vi "Format Class List Table.vi"(5 "Detail Level":T1, 7 "Msg Chain in":string, 8 "error in (no error)":errorcluster, 10 "Class Info Array":T2[](array[typedef]), 11 "VIDoc Printer - Confluence In":refnum<class "VIDoc Printer - Confluence.lvclass">) -> (0 "error out":errorcluster, 2 "Table Text":string, 3 "VIDoc Printer - Confluence Out":refnum<class "VIDoc Printer - Confluence.lvclass">)   [LabVIEW 2023, in "VIDoc Printer - Confluence.lvlib" / "VIDoc Printer - Confluence.lvclass"]
uses:
  VIDoc Printer - Confluence.lvclass
  C:/projects/DMC/Tooling/Git-Action-Service/Source/Documentation Generation/Printers/Printer/VIDoc Printer.lvclass
  Parsing/TypeDefs/Base Class Info Cluster.ctl
  <vilib>/picture/picture.llb/imagedata.ctl
  Settings/Printer Settings/Detail Level Enum.ctl
  VIDoc Printer - Confluence.lvclass/VIDoc Printer - Confluence.ctl
  Accessors/Get Class Column Ordering - Full.vi
  Accessors/Get Class Column Ordering - Minimal.vi
  Accessors/Get Class Column Ordering - Standard.vi
  Accessors/Get Sortable Tables.vi
  Printer/VIDoc Printer.lvclass
  UI Interaction/UI Interaction.lvclass
  Confluence Formatting/Confluence Formatting.lvlib
  C:/projects/DMC/Tooling/Git-Action-Service/Source/Documentation Generation/Printers/Confluence Printer/VIDoc Printer - Confluence.lvclass
  Parsing/VIDoc Parsing.lvlib
  Settings/Printer Settings/Printer Settings.lvclass
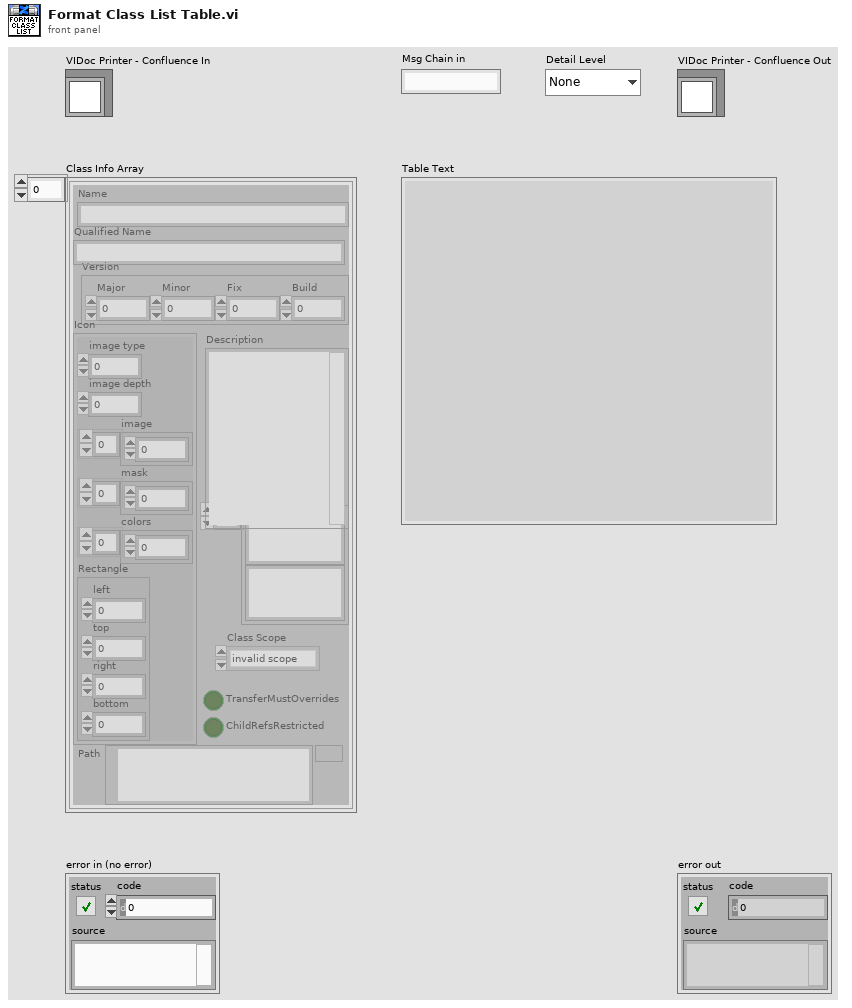
[diagram p1: front panel]
types:
  T1 = typedef "VIDoc Printer.lvlib/Printer Settings.lvclass/Detail Level Enum.ctl" = enum16{"None", "Minimal", "Standard", "Full"}
  T2 = typedef "VIDoc Parsing.lvlib/Base Class Info Cluster.ctl" = cluster{"Name":string, "Icon":T3, "Version":cluster{"Major":u16, "Minor":u16, "Fix":u16, "Build":u16}, "Description":string, "Friends":string[], "ChildRefsRestricted":bool, "TransferMustOverrides":bool, "Path":path, "Qualified Name":string, "Class Scope":enum32{"invalid scope", "public", "private", "protected", "community"}}
  T3 = typedef "imagedata.ctl" = cluster{"image type":i32, "image depth":i32, "image":u8[], "mask":u8[], "colors":u32[], "Rectangle":cluster{"left":i16, "top":i16, "right":i16, "bottom":i16}}
  T4 = cluster{"Major":u16, "Minor":u16, "Fix":u16, "Build":u16}
  T5 = typedef "VIDoc Printer - Confluence.lvlib/VIDoc Settings - Confluence.lvclass/Class Info Column.ctl" = enum16{"Image", "Name", "Description", "Version", "Last Change", "Author", "Commit Hash", "Branch", "Qualified Name", "TransferMustOverrides", "ChildRefsRestricted"}
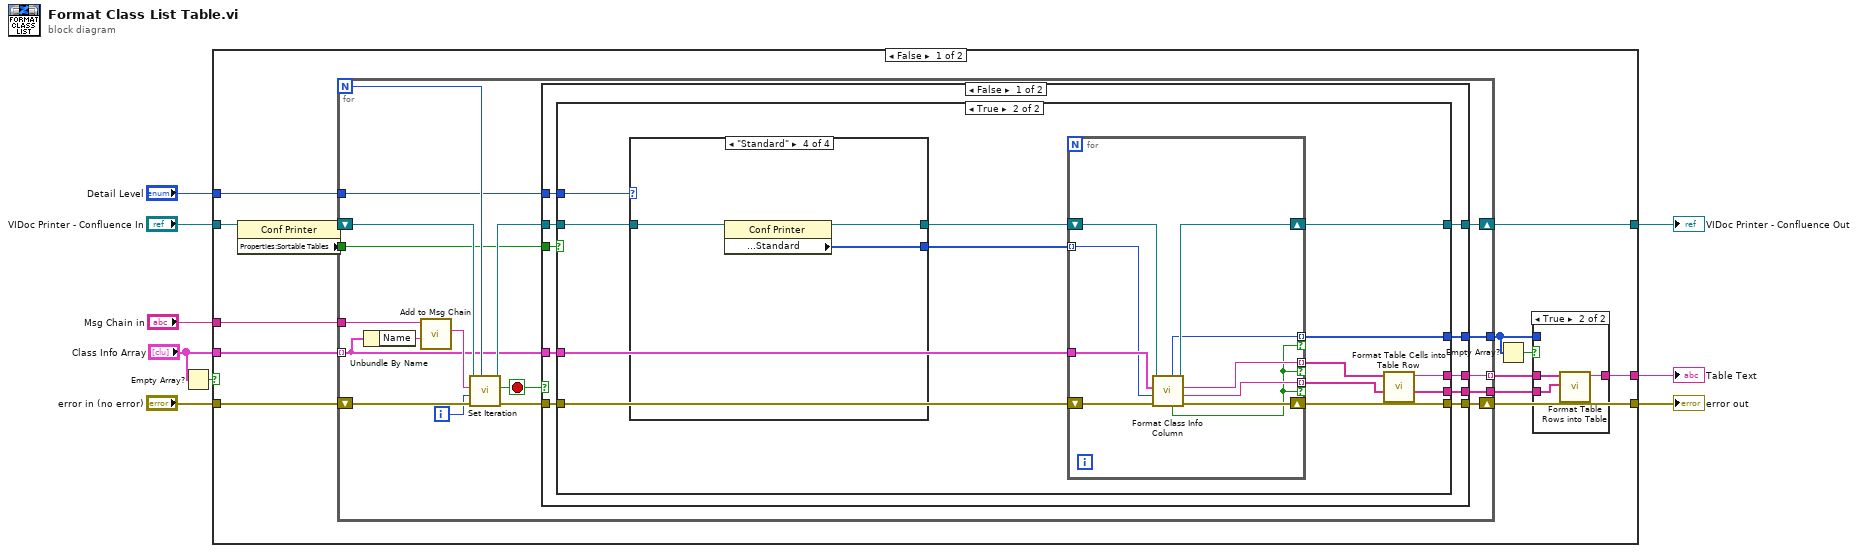
[diagram p0: block diagram]
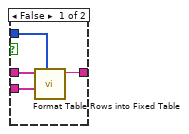
[diagram p2: hidden frame]
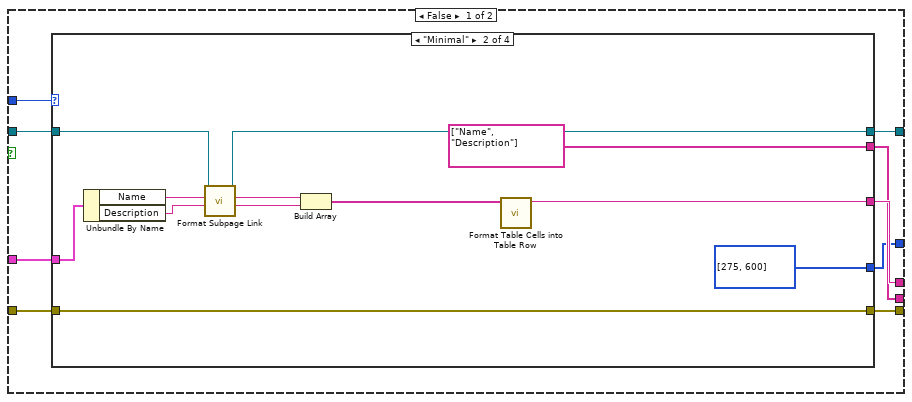
[diagram p3: hidden frame]
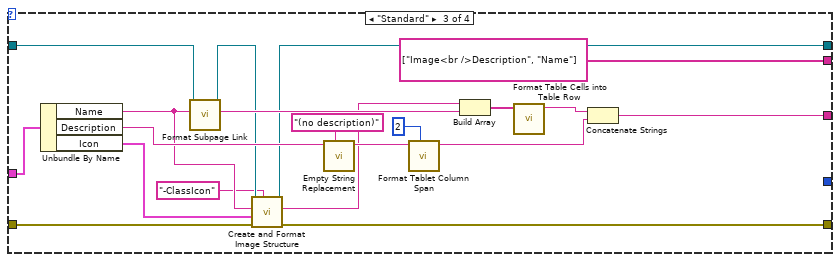
[diagram p5: hidden frame]
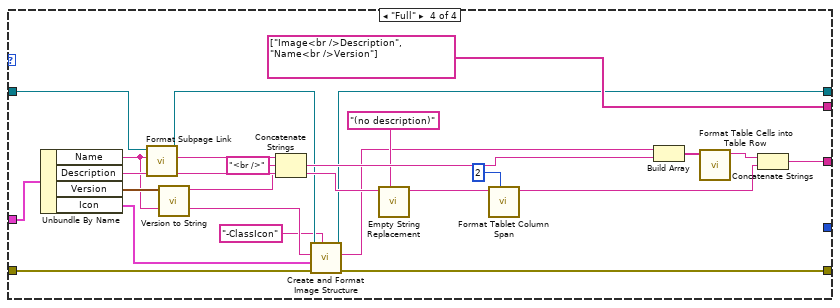
[diagram p6: hidden frame]
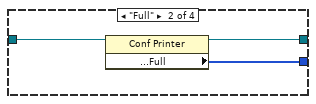
[diagram p8: hidden frame]
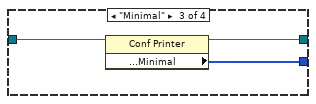
[diagram p9: hidden frame]
diagram:
  n1 = Empty Array?(array="Class Info Array") -> (empty?=w3:bool)
  n2 = case shown="False" w3 {
    tunnel: [w23 w159] -> w9
    tunnel: [w14 _] -> w8
    tunnel: [w22 w160] -> w7
    tunnel: "VIDoc Printer - Confluence In" -> [w18 w160]
    tunnel: "error in (no error)" -> [w21 w159]
    tunnel: "Class Info Array" -> [w20 _]
    tunnel: "Msg Chain in" -> [w19 _]
    tunnel: "Detail Level" -> [w17 _]
    frame False {
      n3 = property class="Conf Printer"(reference=w18) -> (reference out=w13:refnum<class "VIDoc Printer - Confluence.lvclass">, "Properties:Sortable Tables"=w12:bool)  [unwired: 1 in, 1 out]
      n4 = for {
        N -> [w46]
        shift-right: [w37] -> w23
        shift-left: w21 -> [w48]
        shift-right: [w39] -> w22
        shift-left: w13 -> [w47]
        tunnel: w20 -> [w34] mode=indexing
        tunnel: w19 -> [w42]
        tunnel: w17 -> [w38]
        tunnel: [w36] -> w16 mode=indexing
        tunnel: [w35] -> w15
        tunnel: [w33] -> w11
        tunnel: w12 -> [w31]
        i -> [w45]
        stop <- w32 stop-if-true
        n5 = Unbundle By Name(w34) -> ("Name"=w44:string)
        n6 = call "Add to Msg Chain.vi"("New"=w44, "Msg Chain in"=w42) -> ("Msg Chain out"=w43:string)  [unwired: 9 in]
        n7 = call "Set Iteration.vi"("Progress Max"=w46, "error in (no error)"=w48, "Progress Value"=w45, "Message (No Message Update)"=w43, "VIDoc Printer In"=w47) -> ("error out"=w41:errorcluster, "Abort?"=w32:bool, "VIDoc Printer Out"=w40:refnum<class "VIDoc Printer - Confluence.lvclass">)  [unwired: 4 in]
        n8 = case shown="False" w32 {
          tunnel: w41 -> [w57 w158]
          tunnel: w40 -> [w56 w157]
          tunnel: [w54 w157] -> w39
          tunnel: w38 -> [w49 _]
          tunnel: [w53 w158] -> w37
          tunnel: [w52 _] -> w36
          tunnel: [w51 _] -> w35
          tunnel: w34 -> [w55 _]
          tunnel: [w50 _] -> w33
          tunnel: w31 -> [w58 _]
          frame False {
            n9 = case shown="True" w58 {
              tunnel: w57 -> [w67 w135]
              tunnel: w56 -> [w65 w126]
              tunnel: w55 -> [w66 w129]
              tunnel: [w64 w132] -> w54
              tunnel: [w63 w130] -> w53
              tunnel: [w62 w136] -> w52
              tunnel: [w61 w134] -> w51
              tunnel: [w60 w131] -> w50
              tunnel: w49 -> [w59 w128]
              frame False {
                n10 = case shown="\"Minimal\"" w59 {
                  tunnel: [_ w76 w96 w120] -> w62
                  tunnel: [w69 w75 w85 w107] -> w63
                  tunnel: w67 -> [w69 w75 w88 w108]
                  tunnel: [w68 w71 w86 w105] -> w64
                  tunnel: w65 -> [w68 w70 w98 w122]
                  tunnel: w66 -> [_ w80 w97 w121]
                  tunnel: [_ string[] ["Name", "Description"] ("Table Headers") string[] ["Image<br />Description", "Name"] ("Table Headers") string[] ["Image<br />Description", "Name<br />Version"] ("Table Headers")] -> w61
                  tunnel: [_ i16[] [275, 600] ("Column Pixel Widths") _ _] -> w60
                  frame "None" {
                  }
                  frame "Minimal" {
                    n11 = Unbundle By Name(w80) -> ("Name"=w79:string, "Description"=w78:string)
                    n12 = call "Format Subpage Link.vi"("Qualified Name"=w79, "VIDoc Printer - Confluence In"=w70) -> ("Linked HTML"=w72:string, "VIDoc Printer - Confluence Out"=w71:refnum<class "VIDoc Printer - Confluence.lvclass">)  [unwired: 7 in, 1 out]
                    n13 = Build Array(w72, w78) -> (w77:string[])
                    n14 = call "Format Table Cells into Table Row.vi"("Table Cells"=w77) -> ("Table Row Text"=w76:string)  [unwired: 10 in]
                  }
                  frame "Standard" {
                    n15 = Unbundle By Name(w97) -> ("Name"=w84:string, "Description"=w100:string, "Icon"=w83:T3)
                    n16 = call "Format Subpage Link.vi"("Qualified Name"=w84, "VIDoc Printer - Confluence In"=w98) -> ("Linked HTML"=w95:string, "VIDoc Printer - Confluence Out"=w87:refnum<class "VIDoc Printer - Confluence.lvclass">)  [unwired: 7 in, 1 out]
                    n17 = call "Create and Format Image Structure.vi"("Name Addition"="-ClassIcon" ("string"), "Error in"=w88, "Image Data"=w83, "Name"=w84, "VIDoc Printer - Confluence In"=w87) -> ("Error out"=w85:errorcluster, "Image Structure Text"=w81:string, "VIDoc Printer - Confluence Out"=w86:refnum<class "VIDoc Printer - Confluence.lvclass">)  [unwired: 3 in, 1 out]
                    n18 = call "Empty String Replacement.vi"("Empty"="(no description)", "String"=w100) -> ("String Out"=w90:string)  [unwired: 9 in]
                    n19 = call "Format Tablet Column Span.vi"("Column Count"=2 ("Row Span (None)"), "Spanned Cell Text"=w90) -> ("Row Text"=w89:string)  [unwired: 9 in]
                    n20 = Build Array(w81, w95) -> (w94:string[])
                    n21 = call "Format Table Cells into Table Row.vi"("Table Cells"=w94) -> ("Table Row Text"=w93:string)  [unwired: 10 in]
                    n22 = Concatenate Strings(w93, w89) -> (w96:string)
                  }
                  frame "Full" {
                    n23 = Unbundle By Name(w121) -> ("Name"=w104:string, "Description"=w124:string, "Version"=w119:T4, "Icon"=w103:T3)
                    n24 = call "Format Subpage Link.vi"("Qualified Name"=w104, "VIDoc Printer - Confluence In"=w122) -> ("Linked HTML"=w117:string, "VIDoc Printer - Confluence Out"=w106:refnum<class "VIDoc Printer - Confluence.lvclass">)  [unwired: 7 in, 1 out]
                    n25 = call "Version to String.vi"("Version"=w119) -> ("String"=w118:string)  [unwired: 10 in]
                    n26 = Concatenate Strings(w117, "<br />" ("string"), w118) -> (w113:string)
                    n27 = call "Create and Format Image Structure.vi"("Name Addition"="-ClassIcon" ("string"), "Error in"=w108, "Image Data"=w103, "Name"=w104, "VIDoc Printer - Confluence In"=w106) -> ("Error out"=w107:errorcluster, "Image Structure Text"=w102:string, "VIDoc Printer - Confluence Out"=w105:refnum<class "VIDoc Printer - Confluence.lvclass">)  [unwired: 3 in, 1 out]
                    n28 = call "Empty String Replacement.vi"("Empty"="(no description)", "String"=w124) -> ("String Out"=w111:string)  [unwired: 9 in]
                    n29 = call "Format Tablet Column Span.vi"("Column Count"=2 ("Row Span (None)"), "Spanned Cell Text"=w111) -> ("Row Text"=w109:string)  [unwired: 9 in]
                    n30 = Build Array(w102, w113) -> (w116:string[])
                    n31 = call "Format Table Cells into Table Row.vi"("Table Cells"=w116) -> ("Table Row Text"=w115:string)  [unwired: 10 in]
                    n32 = Concatenate Strings(w115, w109) -> (w120:string)
                  }
                }
              }
              frame True {
                n33 = case shown="\"Standard\"" w128 {
                  tunnel: [_ w138 w141 w144] -> w127
                  tunnel: w126 -> [w137 w140 w143 w146]
                  tunnel: [w137 w139 w142 w145] -> w125
                  frame "None" {
                  }
                  frame "Full" {
                    n34 = property class="Conf Printer"(reference=w140) -> (reference out=w139:refnum<class "VIDoc Printer - Confluence.lvclass">, "Properties:Table Column Ordering:Class:Full"=w138:T5[])  [unwired: 1 in, 1 out]
                  }
                  frame "Minimal" {
                    n35 = property class="Conf Printer"(reference=w143) -> (reference out=w142:refnum<class "VIDoc Printer - Confluence.lvclass">, "Properties:Table Column Ordering:Class:Minimal"=w141:T5[])  [unwired: 1 in, 1 out]
                  }
                  frame "Standard" {
                    n36 = property class="Conf Printer"(reference=w146) -> (reference out=w145:refnum<class "VIDoc Printer - Confluence.lvclass">, "Properties:Table Column Ordering:Class:Standard"=w144:T5[])  [unwired: 1 in, 1 out]
                  }
                }
                n37 = for {
                  shift-right: [w155] -> w130
                  shift-left: w135 -> [w156]
                  tunnel: [w154] -> w134 mode=indexing if=w147
                  tunnel: [w153] -> w133 mode=indexing if=w147
                  shift-right: [w151] -> w132
                  shift-left: w125 -> [w152]
                  tunnel: [w150] -> w131 mode=indexing if=w147
                  tunnel: w129 -> [w149]
                  tunnel: w127 -> [w148] mode=indexing
                  n38 = call "Format Class Info Column.vi"("error in (no error)"=w156, "Column"=w148, "Class_Library"=w149, "VIDoc Printer - Confluence In"=w152) -> ("error out"=w155:errorcluster, "Header"=w154:string, "Cell Text"=w153:string, "VIDoc Printer - Confluence Out"=w151:refnum<class "VIDoc Printer - Confluence.lvclass">, "Viable Value?"=w147:bool, "Pixel Width"=w150:i16)  [unwired: 2 in]
                }
                n39 = call "Format Table Cells into Table Row.vi"("Table Cells"=w133) -> ("Table Row Text"=w136:string)  [unwired: 10 in]
              }
            }
          }
          frame True {
          }
        }
      }
      n40 = Empty Array?(array=w11) -> (empty?=w10:bool)
      n41 = case shown="True" w10 {
        tunnel: w16 -> [w27 w30]
        tunnel: w15 -> [w26 w29]
        tunnel: [w25 w28] -> w14
        tunnel: w11 -> [w24 _]
        frame False {
          n42 = call "Format Table Rows into Fixed Table.vi"("Column Pixel Widths"=w24, "Table Headers"=w26, "Table Rows"=w27) -> ("Table Text"=w25:string)  [unwired: 8 in]
        }
        frame True {
          n43 = call "Format Table Rows into Table.vi"("Table Headers"=w29, "Table Rows"=w30) -> ("Table Text"=w28:string)  [unwired: 9 in]
        }
      }
    }
    frame True {
    }
  }
  "error out" <- w9
  "Table Text" <- w8
  "VIDoc Printer - Confluence Out" <- w7
